vi "703_puissance_cor.vi"() -> ()   [LabVIEW 2010]
panel:
  out "Alarme":bool
  out "Voyant":bool
  in  "Marche":bool
  out "Puissance en W":dbl(knob) scale=0.0..1.0 scale format="%.2f"
  in  "Intensité saisie en mA":dbl(slide) scale=0.0..100.0
  in  "R en Ohm":u32
  # "Arrêt"
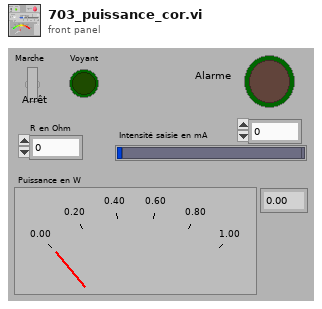
[diagram p1: front panel]
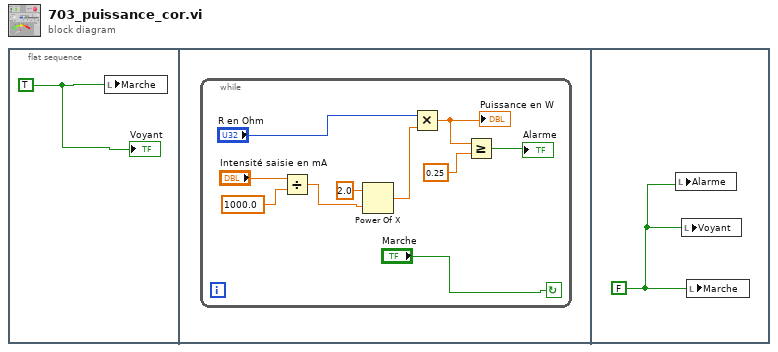
[diagram p0: block diagram]
diagram:
  n1 = flat-sequence {
    frame #0 {
      w1 = TRUE ("Marche")
      n2 = local write "Marche"(w1) -> ()
      "Voyant" <- w1
    }
    frame #1 {
      n3 = while {
        stop <- "Marche" continue-if-true
        n4 = Divide(x="Intensité saisie en mA", y=1000.0) -> (x/y=w3:dbl)
        n5 = Power Of X(1:w3, 2:2.0 ("y")) -> (0:w4:dbl)
        n6 = Multiply(x="R en Ohm", y=w4) -> (x*y=w9:dbl)
        "Puissance en W" <- w9
        n7 = Greater Or Equal?(x=w9, y=0.25) -> (x >= y?=→"Alarme":bool)
      }
    }
    frame #2 {
      w12 = FALSE ("Marche")
      n8 = local write "Alarme"(w12) -> ()
      n9 = local write "Voyant"(w12) -> ()
      n10 = local write "Marche"(w12) -> ()
    }
  }
